vi "CRUD Delete Example.vi"() -> ()   [LabVIEW 2020, in "ORM_Examples.lvlib"]
doc: "This performs a DELETE operation on the table corresponding to the bbPlayers class based on the value of the primary key (playerNum) provided as an input. affectedRows returns the number of rows that were deleted. This also uses BB Players Map class."
uses:
  ORM_Examples.lvlib
  BB Players/bbPlayers.lvclass
  BB Players Map/BB Players Map.lvclass
  C:/Program Files/National Instruments/LabVIEW 2024/vi.lib/Viviota/shared/ORM.lvlibp/ORM/TypeMap/TypeMap.lvclass
  C:/Program Files/National Instruments/LabVIEW 2024/vi.lib/Viviota/shared/ORM.lvlibp/Transaction Logger/Log Map/LogMap.lvclass
  97c0ae94-fa72-4a2f-a348-d9eb05801b12.vi
  97c0ae94-fa72-4a2f-a348-d9eb05801b12.vi/93c2cd5d-a53a-4cc2-b8c3-9c3eef6598b6.vi
  <vilib>/Viviota/shared/ORM_ADONet.lvlibp/ADOMapper/ADOMapper.lvclass
  C:/Program Files/National Instruments/LabVIEW 2024/vi.lib/Viviota/shared/ORM.lvlibp/ORM/SqlMapper/SqlMapper.lvclass
  <vilib>/Viviota/shared/ORM.lvlibp/ORM/TypeMap/Write Autokey.vi
  <vilib>/Viviota/shared/ORM.lvlibp/ORM/TypeMap/Write Table Name.vi
  <vilib>/Viviota/shared/ORM.lvlibp/Transaction Logger/Log Map/Write Log Table Name.vi
  <vilib>/Viviota/shared/ORM_DBC_Sqlite.lvlibp/Sqlite Connect.vi
  <vilib>/Utility/error.llb/Error Cluster From Error Code.vi
  <vilib>/Viviota/shared/ORM.lvlibp/ORM/TypeMap/Read TypeMap.vi
  <vilib>/Viviota/shared/ORM.lvlibp/ORM/SqlMapper/End Transaction.vi
  <vilib>/Viviota/shared/ORM.lvlibp/ORM/TypeMap/TypeMap.lvclass
  ORM_API/ORM_API.lvlib
  <vilib>/Viviota/shared/ORM_ADONet.lvlibp
  <vilib>/Viviota/shared/ORM_DBC_Sqlite.lvlibp/DBC.lvclass
  C:/Program Files/National Instruments/LabVIEW 2024/vi.lib/Viviota/shared/ORM_ADONet.lvlibp/ADOMapper/ADOMapper.lvclass
panel:
  out "affectedRows":i32
  in  "playerNum":i32
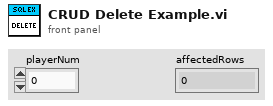
[diagram p1: front panel]
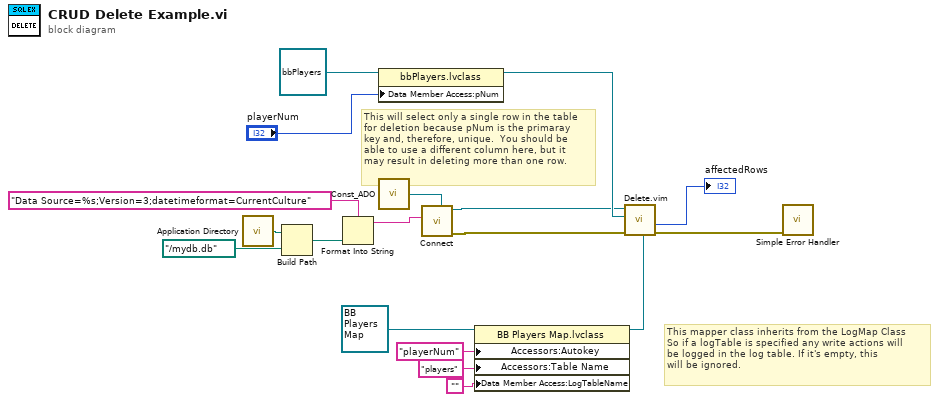
[diagram p0: block diagram]
diagram:
  # "This mapper class inherits from the LogMap Class\nSo if a logTable is specified any write actions will\nbe logged in the log table. If it's empty, this \nwill be ignored."
  # "This will select only a single row in the table\nfor deletion because pNum is the primaray\nkey and, therefore, unique.  You should be\nable to use a different column here, but it\nmay result in deleting more than one row."
  n1 = call <vilib>:"Application Directory.vi"() -> ("Application Directory"=w7:path)
  n2 = Build Path(base path=w7, name or relative path=path "../mydb.db" ("file out")) -> (appended path=w8:path)
  n3 = Format Into String(format string="Data Source=%s;Version=3;datetimeformat=CurrentCulture" ("connectionStringName"), w8) -> (resulting string=w3:string)  [unwired: 2 in, 1 out]
  n4 = property class="bbPlayers.lvclass"(reference=refnum<class "bbPlayers.lvclass"> refnum ("bbPlayers.lvclass"), "Data Member Access:pNum"="playerNum") -> (reference out=w15:refnum<class "bbPlayers.lvclass">)  [unwired: 1 in, 1 out]
  n5 = call <vilib>:"Const_ADO.vi"() -> ("ADOMapper"=w4:refnum<class "ADOMapper.lvclass">)
  n6 = call-poly "Connect.vi"("SqlMapper Type"=w4, "Connection String"=w3) -> ("error out"=w1:errorcluster, "SqlMapper out"=w2:refnum<class "ADOMapper.lvclass">)  [unwired: 8 in]
  n7 = property class="BB Players Map.lvclass"(reference=refnum<class "BB Players Map.lvclass"> refnum ("BB Players Map.lvclass"), "Accessors:Autokey"="playerNum" ("Autokey"), "Accessors:Table Name"="players" ("Table Name"), "Data Member Access:LogTableName"="") -> (reference out=w13:refnum<class "BB Players Map.lvclass">)  [unwired: 1 in, 1 out]
  n8 = call "Delete.vim"("TypeMap in"=w13, "error in (no error)"=w1, "object in"=w15, "SqlMapper in"=w2) -> ("error out"=w18:errorcluster, "affectedRows"=→"affectedRows":i32)  [unwired: 5 in, 1 out]
  n9 = call <vilib>:"Simple Error Handler.vi"("error in (no error)"=w18) -> ()  [unwired: 4 in, 5 out]
